vi "Get Output Range.vi"(8 "error in (no error)":errorcluster, 11 "VISA resource name":refnum<visa-resource-name>) -> (0 "error out":errorcluster, 1 "Secondary Output":string, 2 "Primary Output":string, 3 "VISA resource name out":refnum<visa-resource-name>)   [LabVIEW 2014, in "Fluke 5XXX Series Multicalibrators.lvlib"]
doc: "This VI the present output ranges. Both the primary output and secondary outputs are returned. If there is no secondary output, 0 is returned.\n\nNote:\n\n(1) Instrument models 5700A and 5720A are not equipped with dual outpus. Only single output operations are available."
uses:
  Fluke 5XXX Series Multicalibrators.lvlib
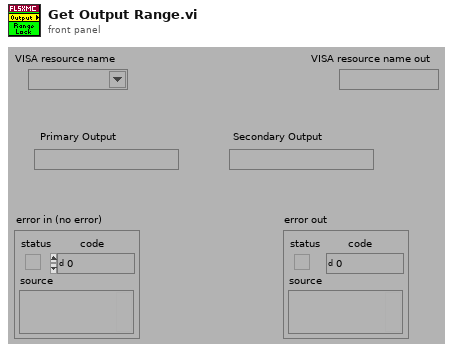
[diagram p1: front panel]
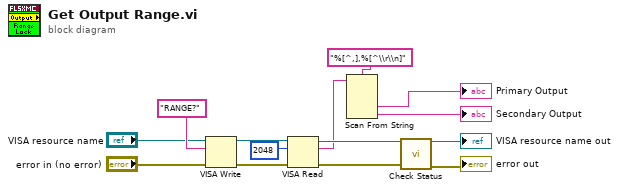
[diagram p0: block diagram]
diagram:
  n1 = VISA Write(VISA resource name="VISA resource name", write buffer="RANGE?", error in (no error)="error in (no error)") -> (VISA resource name out=w13:refnum<visa-resource-name>, error out=w12:errorcluster)  [unwired: 1 out]
  n2 = VISA Read(VISA resource name=w13, byte count=u32 2048 ("byte count (0)"), error in (no error)=w12) -> (VISA resource name out=w8:refnum<visa-resource-name>, read buffer=w2:string, error out=w9:errorcluster)  [unwired: 1 out]
  n3 = Scan From String(format string="%[^,],%[^\\r\\n]", input string=w2) -> (output 1=→"Primary Output":string, output 2=→"Secondary Output":string)  [unwired: 4 in, 3 out]
  n4 = call "Check Status.vi"("VISA resource name"=w8, "error in (no error)"=w9) -> ("VISA resource name out"=→"VISA resource name out":refnum<visa-resource-name>, "error out"=→"error out":errorcluster)  [unwired: 12 in]
